vi "Persistent.vi"(8 "error in":T1, 10 "Persistent":bool, 11 "VISA Resource Name":refnum<visa-resource-name>="TCPIP0::10.0.0.1::7185::SOCKET") -> (0 "error out":T1, 3 "VISA Resource Name Out":refnum<visa-resource-name>)   [LabVIEW 2019]
uses:
  Persistent States.ctl
panel:
  out "Magnet Voltage retries":i16
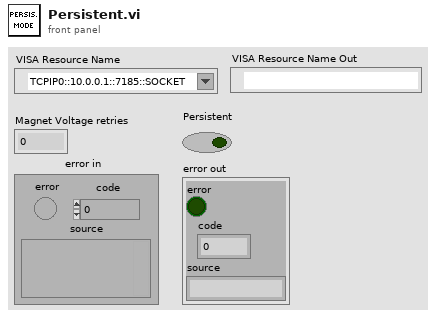
[diagram p1: front panel]
types:
  T1 = cluster{"error":bool, "code":i32, "source":string}
  T2 = typedef "Persistent States.ctl" = enum16{"Initialize", "Check Heater", "Check Mode Enter", "Check Magnet Voltage Enter", "Cool Switch", "Check Mode Exit", "Check Magnet Current Exit", "Heat Switch", "Stop"}
  T3 = enum16{"", "RAMPING", "HOLDING", "PAUSED", "MANUAL UP", "MANUAL DOWN", "ZEROING CURRENT", "QUENCH DETECTED", "AT ZERO", "HEATING SWITCH", "COOLING SWITCH", "EXTERNAL RAMPDOWN"}
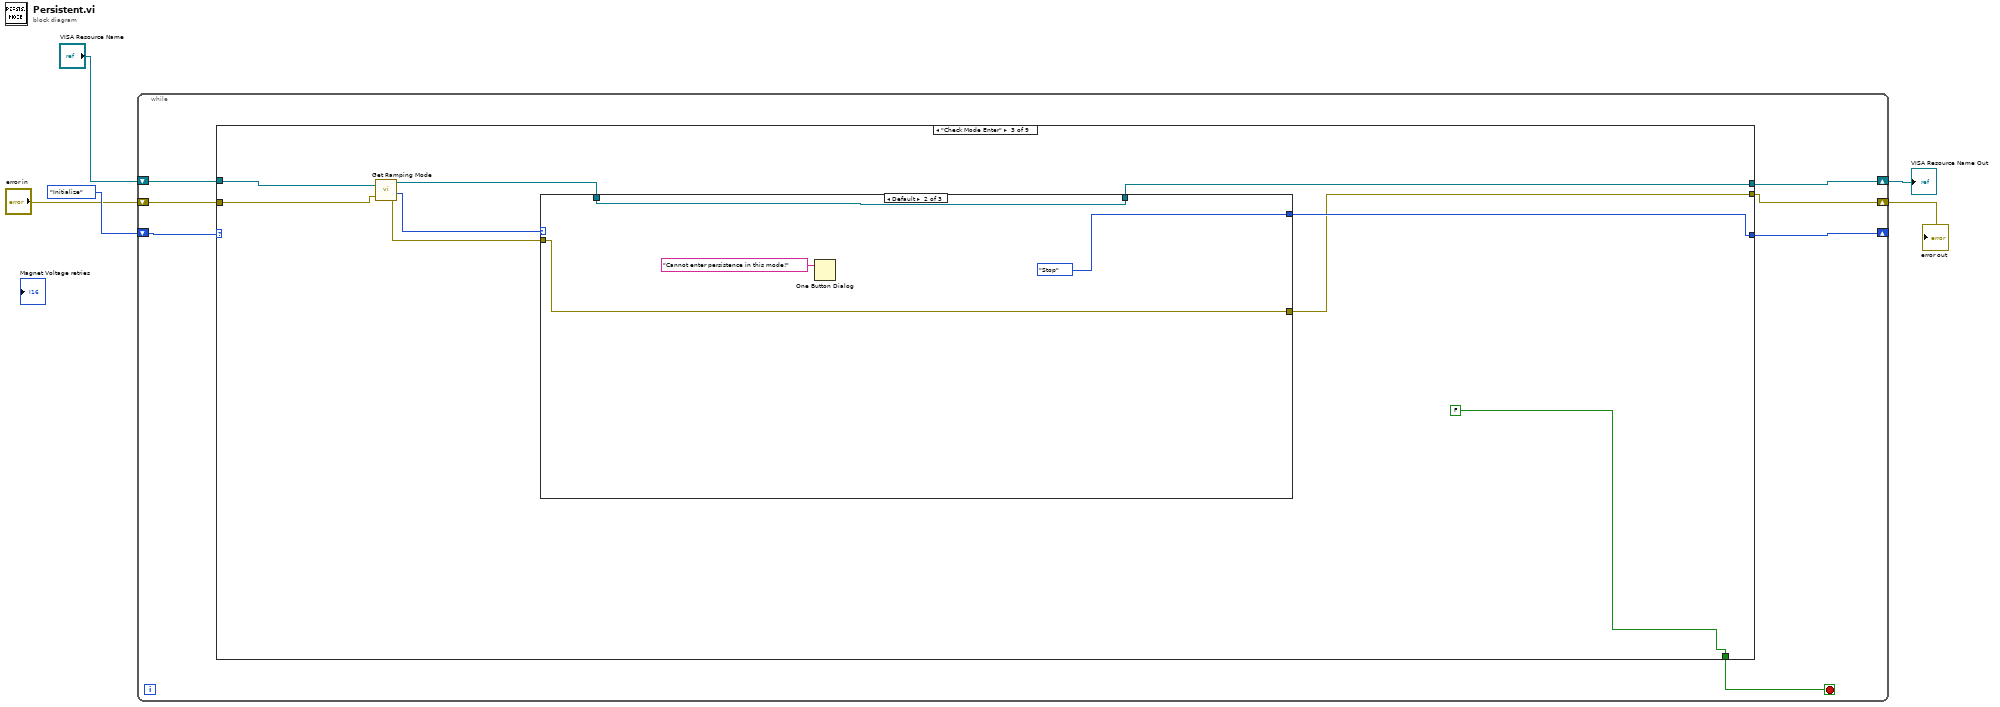
[diagram p0: block diagram]
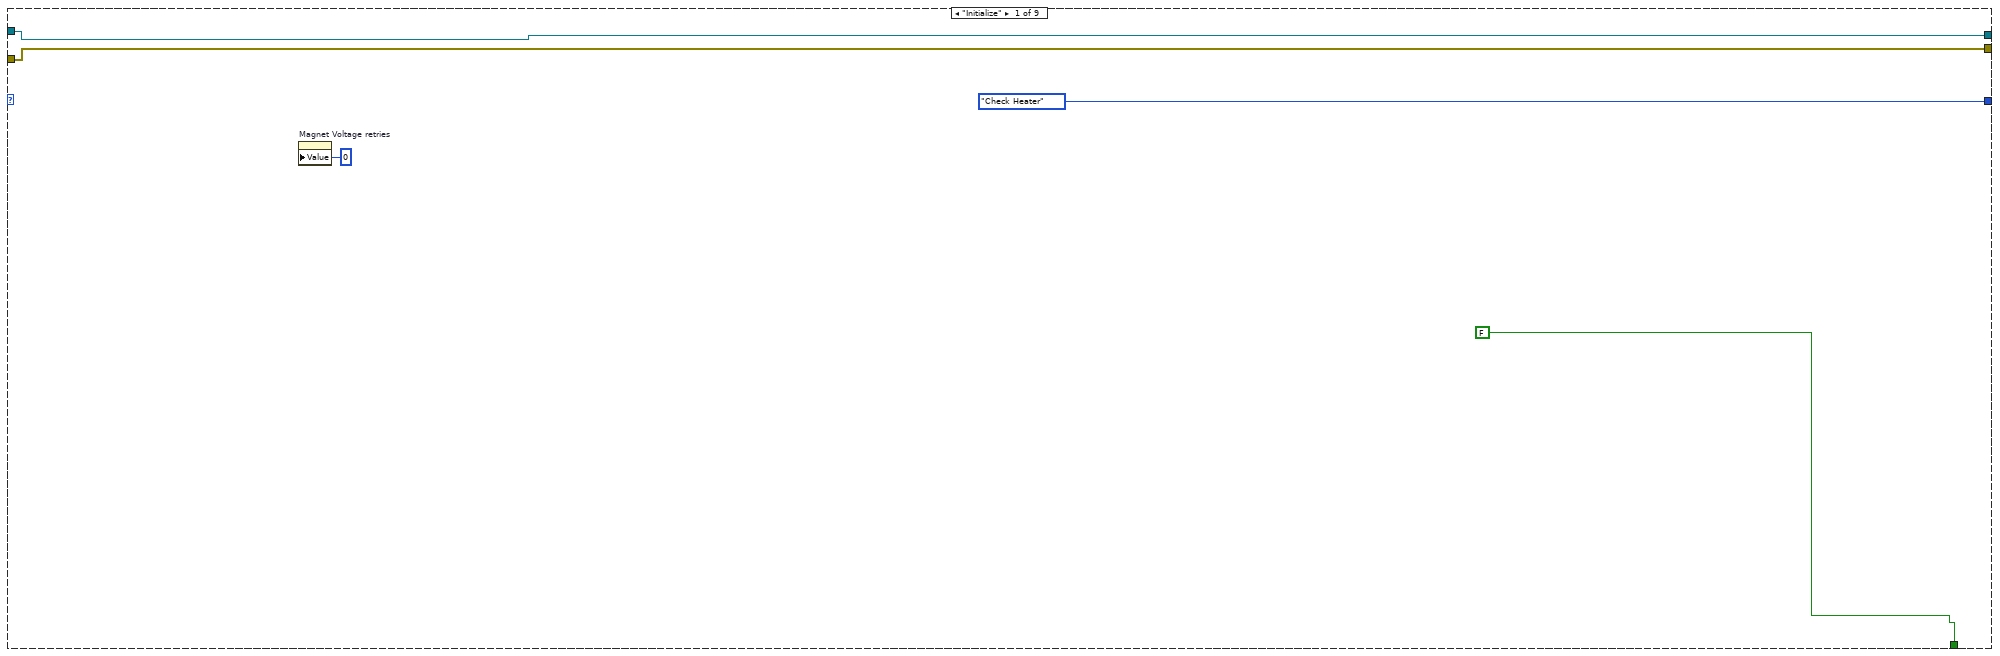
[diagram p2: hidden frame]
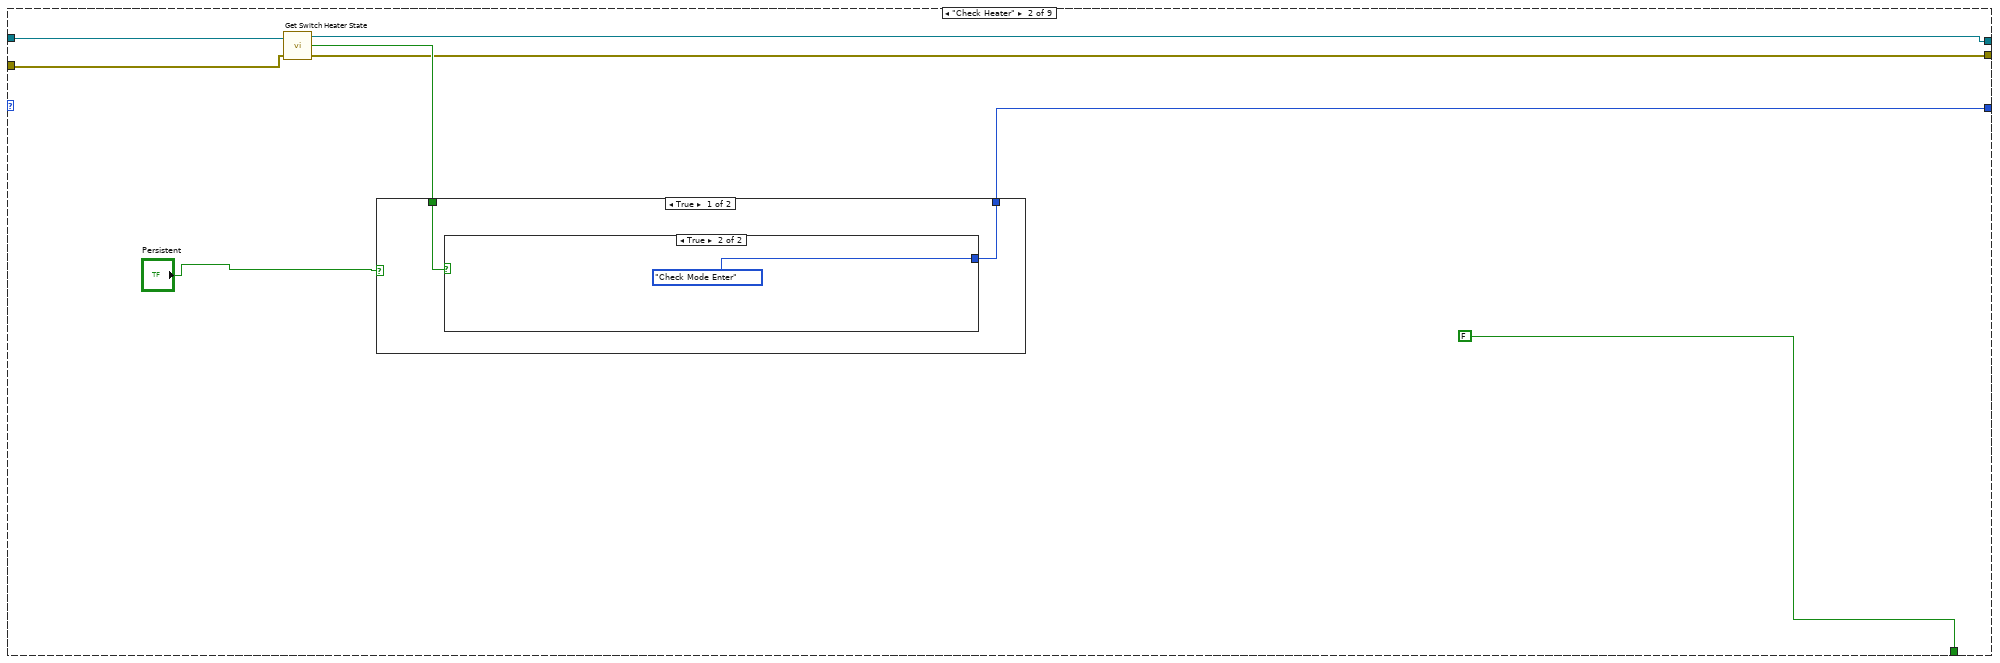
[diagram p3: hidden frame]
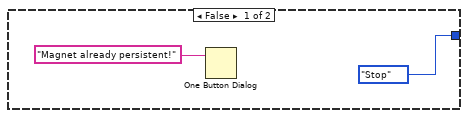
[diagram p4: hidden frame]
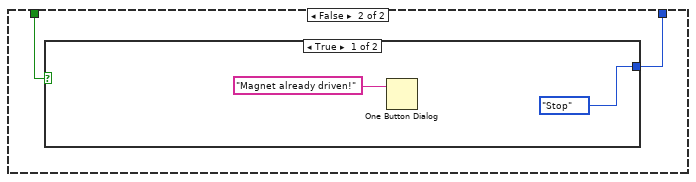
[diagram p5: hidden frame]
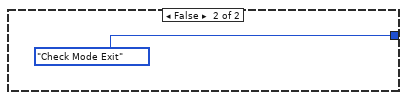
[diagram p6: hidden frame]
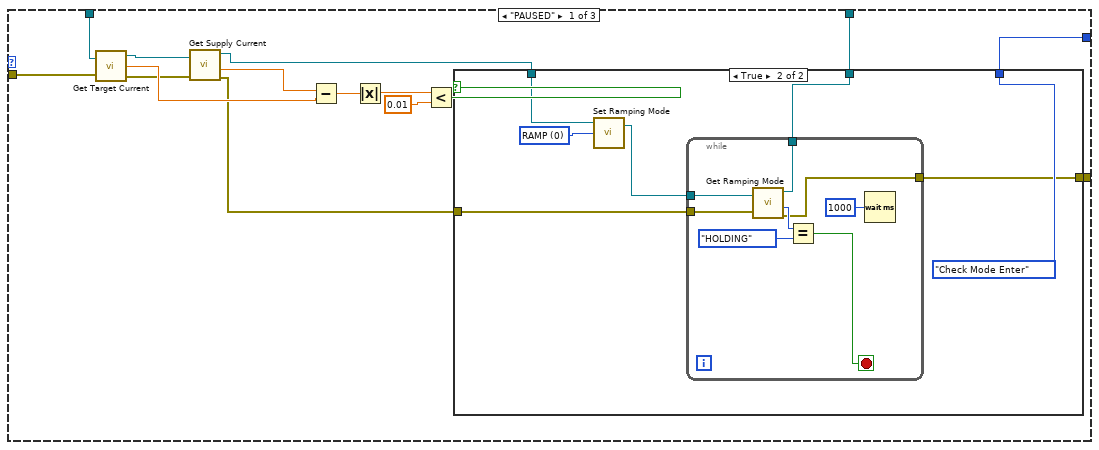
[diagram p7: hidden frame]
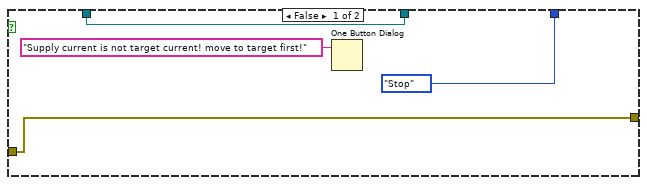
[diagram p8: hidden frame]
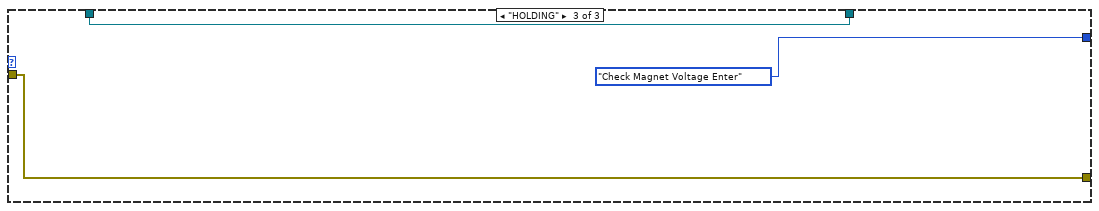
[diagram p9: hidden frame]
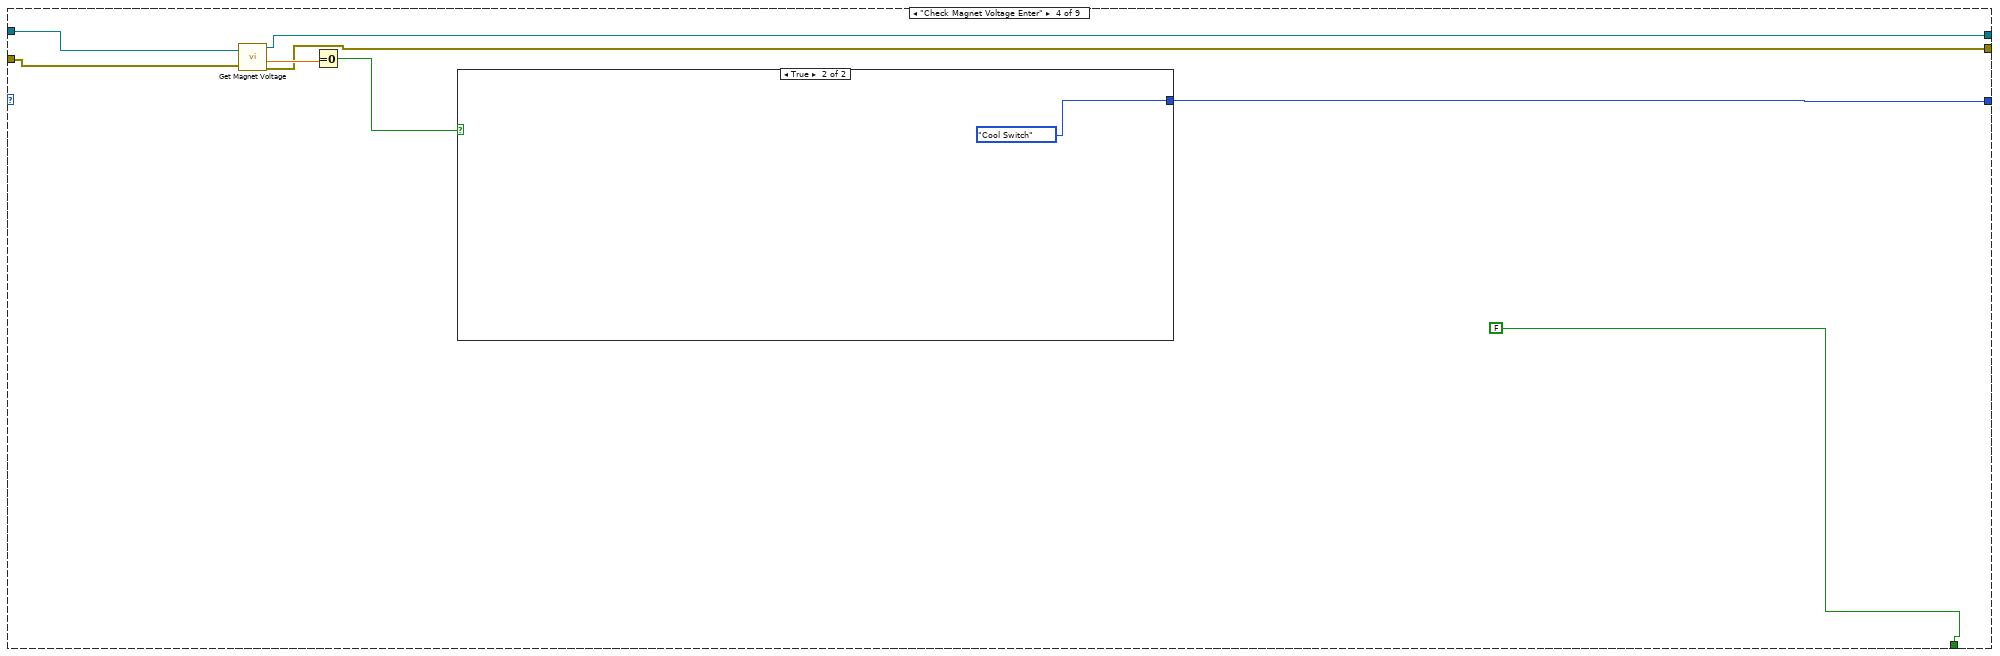
[diagram p10: hidden frame]
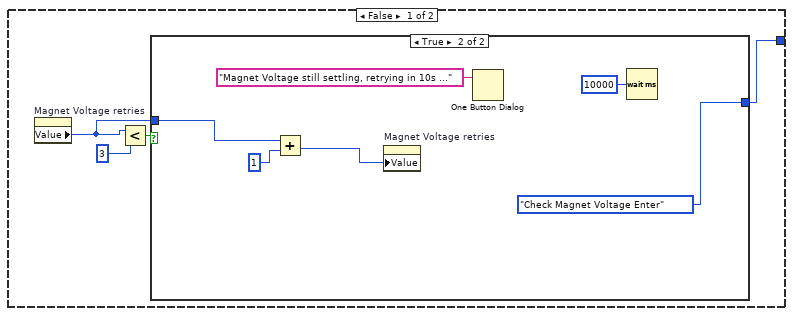
[diagram p11: hidden frame]
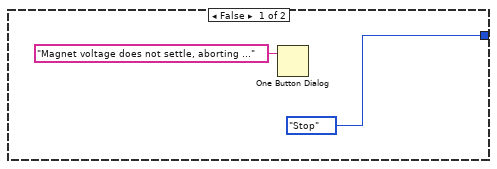
[diagram p12: hidden frame]
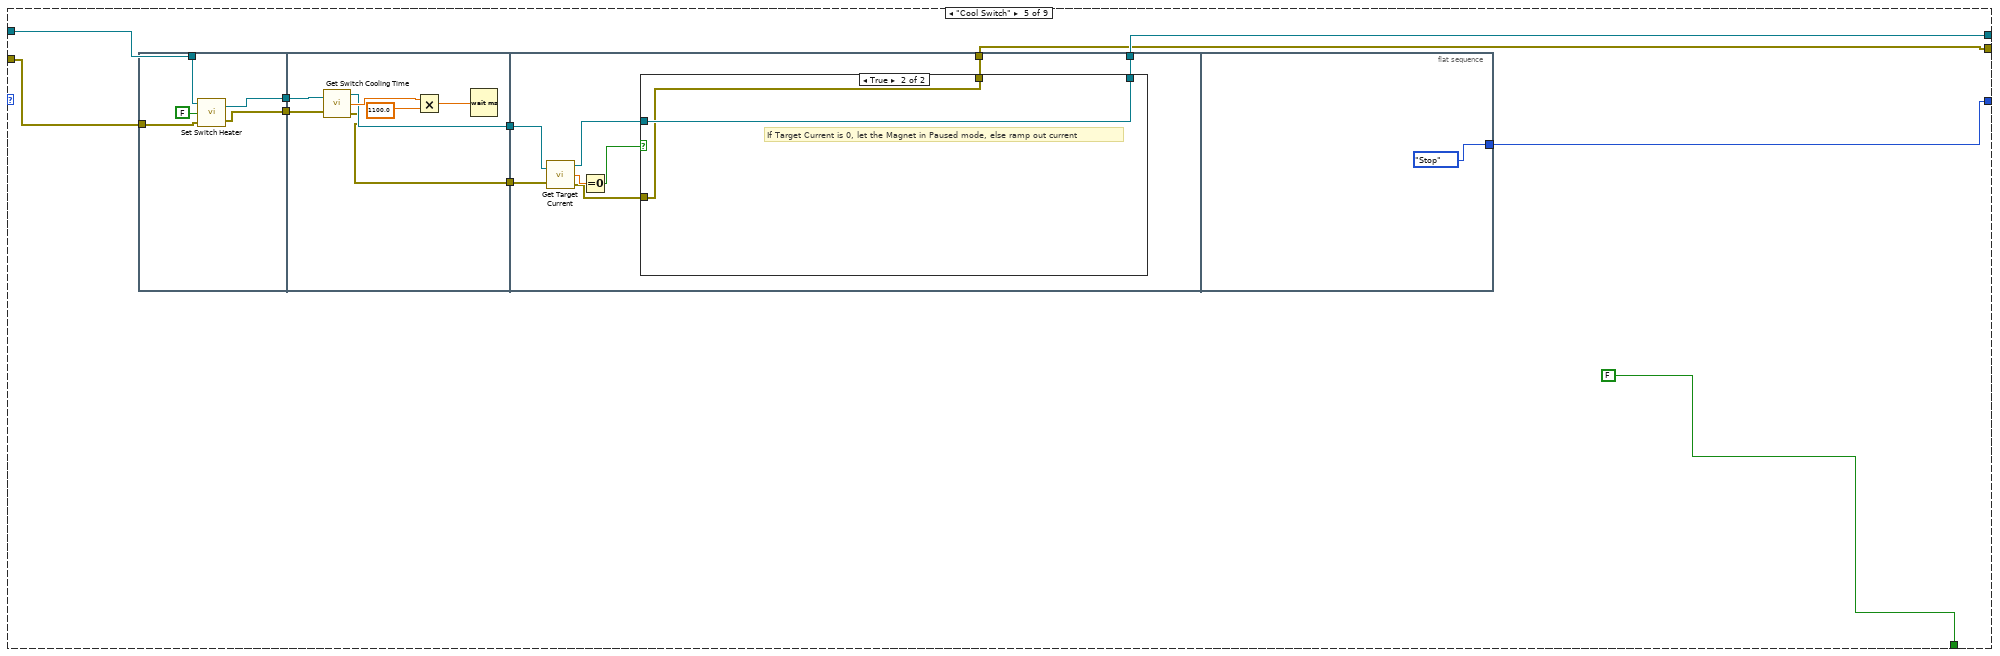
[diagram p13: hidden frame]
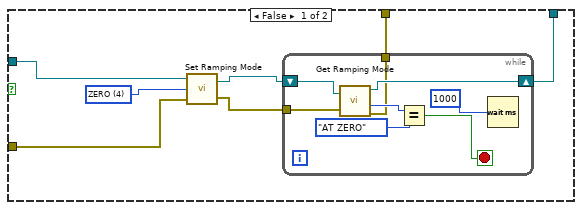
[diagram p14: hidden frame]
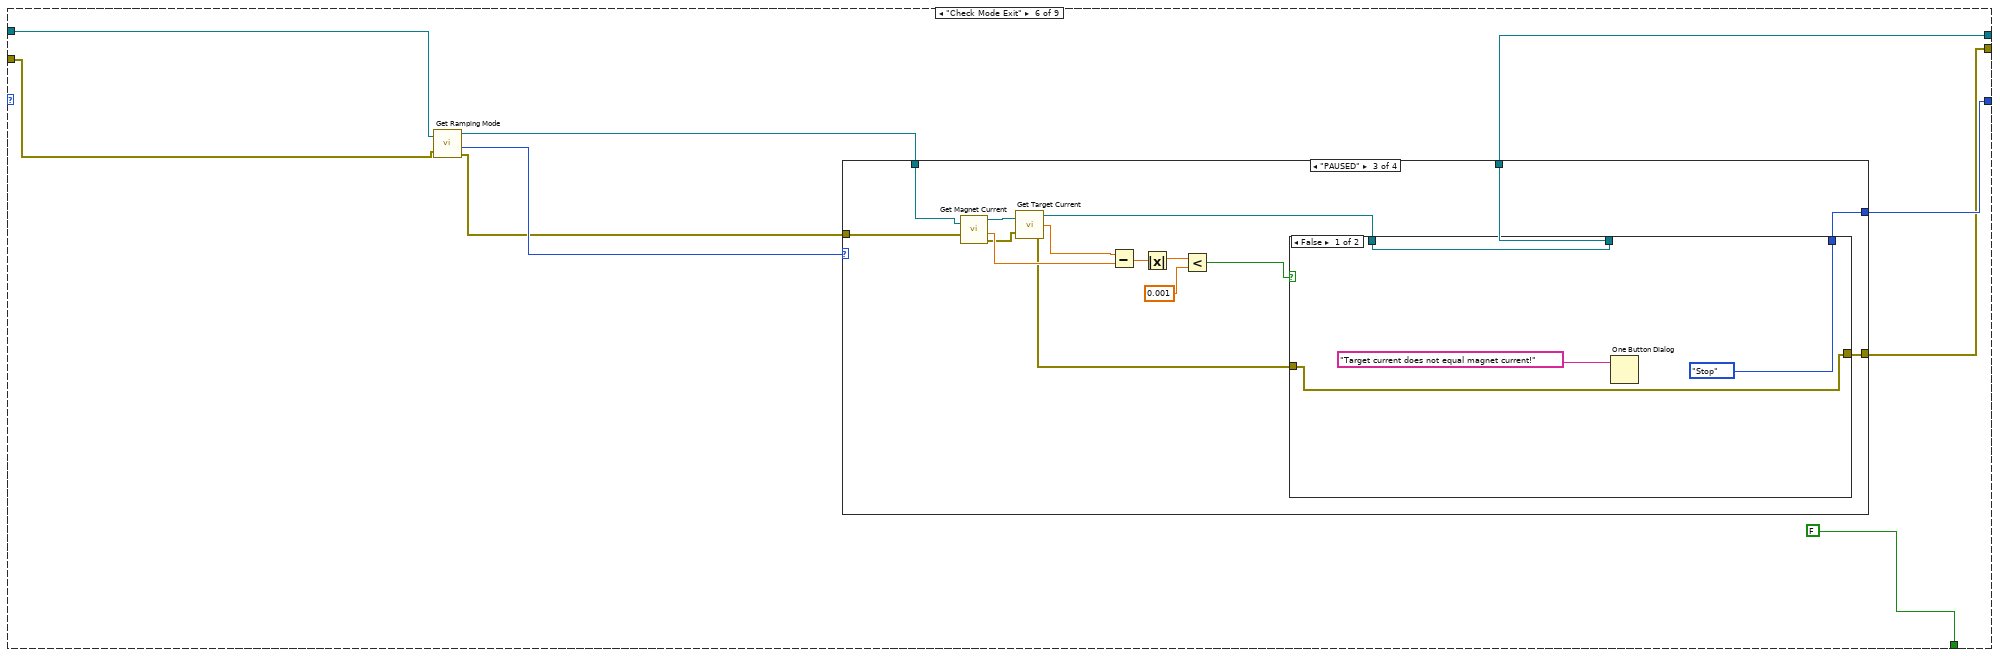
[diagram p15: hidden frame]
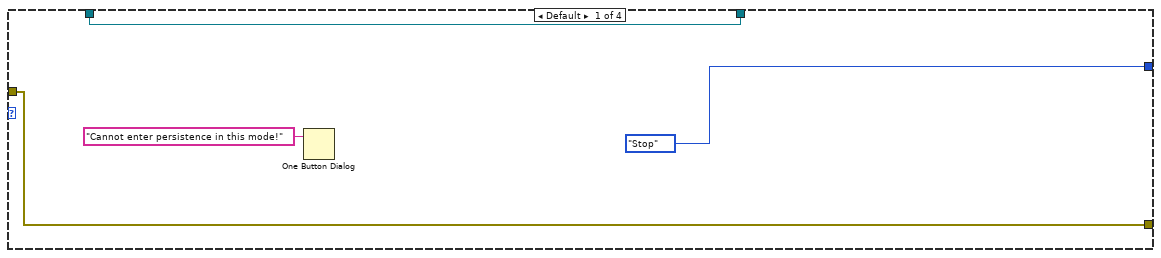
[diagram p16: hidden frame]
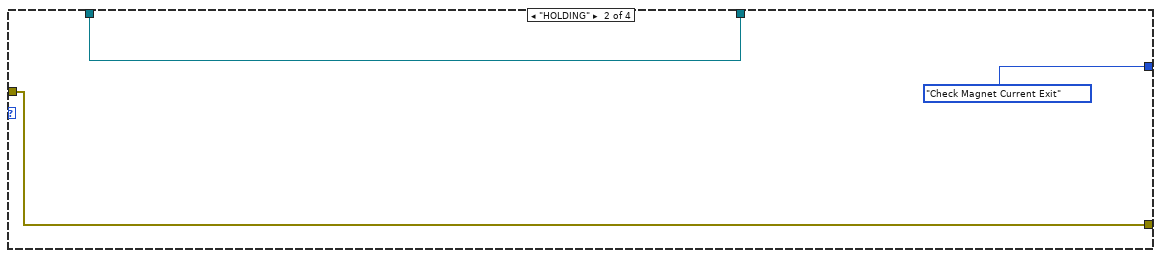
[diagram p17: hidden frame]
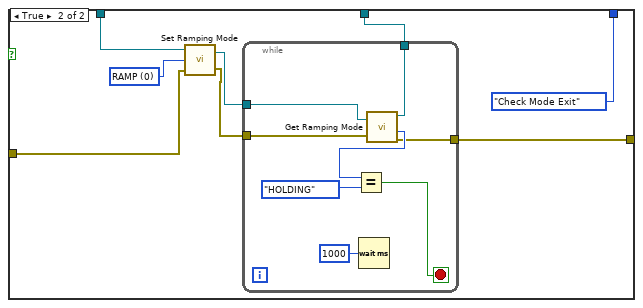
[diagram p18: hidden frame]
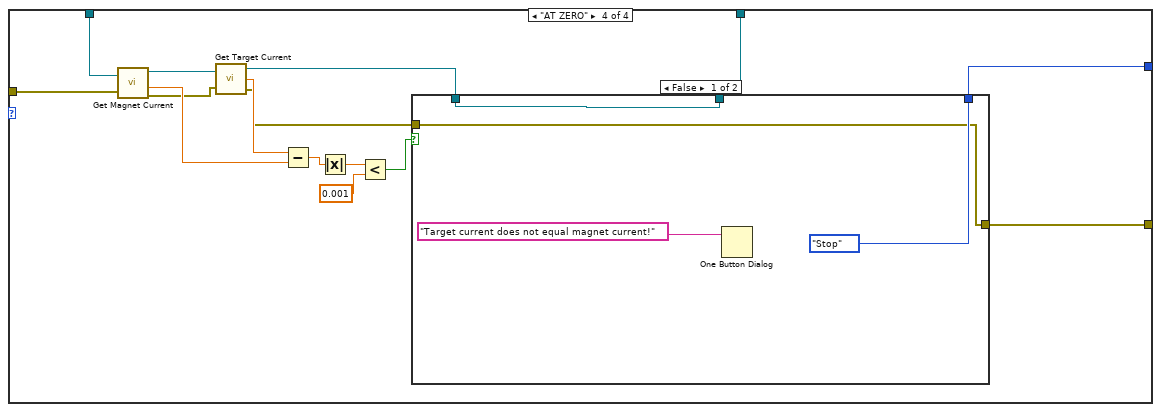
[diagram p19: hidden frame]
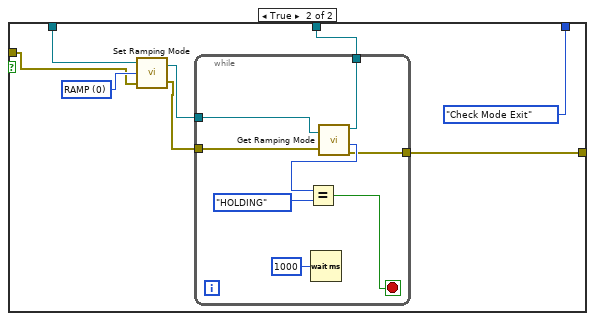
[diagram p20: hidden frame]
diagram:
  n1 = while {
    shift-right: [w10] -> _
    shift-left: Persistent_States."Initialize" -> [w12]
    shift-right: [w11] -> w3
    shift-left: "VISA Resource Name" -> [w9]
    shift-right: [w6] -> w1
    shift-left: "error in" -> [w7]
    stop <- w8 stop-if-true
    n2 = case shown="\"Check Mode Enter\"" w12 {
      tunnel: [w14 w24 w41 w92 w111 w159 w245 w262 w281] -> w11
      tunnel: [Persistent_States."Check Heater" w21 w40 w89 w113 w161 w246 w263 Persistent_States."Stop"] -> w10
      tunnel: w9 -> [w14 w25 w44 w93 w116 w163 w254 w265 w281]
      tunnel: [FALSE FALSE FALSE FALSE FALSE FALSE FALSE FALSE TRUE] -> w8
      tunnel: w7 -> [w13 w19 w38 w87 w110 w157 w243 w260 w279]
      tunnel: [w13 w18 w36 w86 w107 w155 w241 w258 w279] -> w6
      frame "Initialize" {
        n3 = property on="Magnet Voltage retries" class="DigNum (strict)"("Value"=i16 0 ("Magnet Voltage retries")) -> ()  [unwired: 2 in, 2 out]
      }
      frame "Check Heater" {
        n4 = call "Get Switch Heater State.vi"("error in"=w19, "VISA resource name"=w25) -> ("error out"=w18:T1, "Switch Heater state"=w22:bool, "VISA resource name out"=w24:refnum<visa-resource-name>)  [unwired: 1 in]
        n5 = case shown="True" "Persistent" {
          tunnel: w22 -> [w27 w32]
          tunnel: [w26 w31] -> w21
          frame True {
            n6 = case shown="True" w27 {
              tunnel: [Persistent_States."Stop" Persistent_States."Check Mode Enter"] -> w26
              frame False {
                n7 = One Button Dialog(message="Magnet already persistent!") -> ()  [unwired: 1 in, 1 out]
              }
              frame True {
              }
            }
          }
          frame False {
            n8 = case shown="True" w32 {
              tunnel: [Persistent_States."Stop" Persistent_States."Check Mode Exit"] -> w31
              frame True {
                n9 = One Button Dialog(message="Magnet already driven!") -> ()  [unwired: 1 in, 1 out]
              }
              frame False {
              }
            }
          }
        }
      }
      frame "Check Mode Enter" {
        n10 = call "Get Ramping Mode.vi"("VISA resource name"=w44, "error in"=w38) -> ("VISA resource name out"=w42:refnum<visa-resource-name>, "Ramping Mode"=w39:T3, "error out"=w37:T1)  [unwired: 1 out]
        n11 = case shown="Default" w39 {
          tunnel: [w51 Persistent_States."Stop" Persistent_States."Check Magnet Voltage Enter"] -> w40
          tunnel: w42 -> [w59 w80 w84]
          tunnel: [w49 w80 w84] -> w41
          tunnel: w37 -> [w48 w79 w83]
          tunnel: [w45 w79 w83] -> w36
          frame "PAUSED" {
            n12 = call "Get Target Current.vi"("VISA resource name"=w59, "error in"=w48) -> ("VISA resource name out"=w58:refnum<visa-resource-name>, "Target Current (A)"=w56:dbl, "error out"=w47:T1)
            n13 = call "Get Supply Current.vi"("VISA resource name"=w58, "error in"=w47) -> ("VISA resource name out"=w50:refnum<visa-resource-name>, "Supply Current (A)"=w57:dbl, "error out"=w46:T1)  [unwired: 1 out]
            n14 = Subtract(x=w57, y=w56) -> (x-y=w55:dbl)
            n15 = Absolute Value(x=w55) -> (abs(x)=w54:dbl)
            n16 = Less?(x=w54, y=0.01) -> (x < y?=w52:bool)
            n17 = case shown="True" w52 {
              tunnel: [Persistent_States."Stop" Persistent_States."Check Mode Enter"] -> w51
              tunnel: w50 -> [w61 w70]
              tunnel: [w61 w66] -> w49
              tunnel: w46 -> [w60 w65]
              tunnel: [w60 w64] -> w45
              frame False {
                n18 = One Button Dialog(message="Supply current is not target current! move to target first!") -> ()  [unwired: 1 in, 1 out]
              }
              frame True {
                w69 = u16 0 items=["RAMP", "PAUSE", "MANUAL UP", "MANUAL DOWN", "ZERO"] ("Ramping Mode")
                n19 = call "Set Ramping Mode.vi"("Ramping Mode"=w69, "VISA resource name"=w70) -> ("VISA resource name out"=w67:refnum<visa-resource-name>)  [unwired: 1 in, 1 out]
                n20 = while {
                  tunnel: w67 -> [w78]
                  tunnel: [w77] -> w66
                  tunnel: w65 -> [w72]
                  tunnel: [w71] -> w64
                  stop <- w74 stop-if-true
                  n21 = call "Get Ramping Mode.vi"("VISA resource name"=w78, "error in"=w72) -> ("VISA resource name out"=w77:refnum<visa-resource-name>, "Ramping Mode"=w76:T3, "error out"=w71:T1)  [unwired: 1 out]
                  n22 = Equal?(x=w76, y=T3."HOLDING") -> (x = y?=w74:bool)
                  n23 = Wait (ms)(milliseconds to wait=u32 1000) -> ()  [unwired: 1 out]
                }
              }
            }
          }
          frame Default {
            n24 = One Button Dialog(message="Cannot enter persistence in this mode!") -> ()  [unwired: 1 in, 1 out]
          }
          frame "HOLDING" {
          }
        }
      }
      frame "Check Magnet Voltage Enter" {
        n25 = call "Get Magnet Voltage.vi"("VISA resource name"=w93, "error in"=w87) -> ("VISA resource name out"=w92:refnum<visa-resource-name>, "Magnet Voltage (V)"=w91:dbl, "error out"=w86:T1)  [unwired: 1 out]
        n26 = Equal To 0?(x=w91) -> (x = 0?=w90:bool)
        n27 = case shown="True" w90 {
          tunnel: [w94 Persistent_States."Cool Switch"] -> w89
          frame False {
            n28 = property on="Magnet Voltage retries" class="DigNum (strict)"() -> ("Value"=w95:i16)  [unwired: 2 in, 2 out]
            n29 = Less?(x=w95, y=i16 3) -> (x < y?=w96:bool)
            n30 = case shown="True" w96 {
              tunnel: w95 -> [_ w105]
              tunnel: [Persistent_States."Stop" Persistent_States."Check Magnet Voltage Enter"] -> w94
              frame False {
                n31 = One Button Dialog(message="Magnet voltage does not settle, aborting ...") -> ()  [unwired: 1 in, 1 out]
              }
              frame True {
                n32 = Add(x=w105, y=i16 1) -> (x+y=w103:i16)
                n33 = property on="Magnet Voltage retries" class="DigNum (strict)"("Value"=w103) -> ()  [unwired: 2 in, 2 out]
                n34 = One Button Dialog(message="Magnet Voltage still settling, retrying in 10s ...") -> ()  [unwired: 1 in, 1 out]
                n35 = Wait (ms)(milliseconds to wait=u32 10000) -> ()  [unwired: 1 out]
              }
            }
          }
          frame True {
          }
        }
      }
      frame "Cool Switch" {
        n36 = flat-sequence {
          tunnel: w116 -> [w120]
          tunnel: [w119] -> w115
          tunnel: w110 -> [w118]
          tunnel: [w117] -> w109
          tunnel: w115 -> [w128]
          tunnel: [w124] -> w114
          tunnel: w109 -> [w123]
          tunnel: [w122] -> w108
          tunnel: w114 -> [w136]
          tunnel: [w132] -> w111
          tunnel: w108 -> [w131]
          tunnel: [w129] -> w107
          tunnel: [Persistent_States."Stop"] -> w113
          frame #0 {
            n37 = call "Set Switch Heater.vi"("error in"=w118, "Switch Heater Control"=FALSE, "VISA resource name"=w120) -> ("error out"=w117:T1, "VISA resource name out"=w119:refnum<visa-resource-name>)
          }
          frame #1 {
            n38 = call "Get Switch Cooling Time.vi"("VISA resource name"=w128, "error in"=w123) -> ("VISA resource name out"=w124:refnum<visa-resource-name>, "Switch Cooling Time (secs)"=w126:dbl, "error out"=w122:T1)
            n39 = Multiply(x=w126, y=1100.0) -> (x*y=w125:dbl)
            n40 = Wait (ms)(milliseconds to wait=w125) -> ()  [unwired: 1 out]
          }
          frame #2 {
            n41 = call "Get Target Current.vi"("VISA resource name"=w136, "error in"=w131) -> ("VISA resource name out"=w133:refnum<visa-resource-name>, "Target Current (A)"=w135:dbl, "error out"=w130:T1)
            n42 = Equal To 0?(x=w135) -> (x = 0?=w134:bool)
            n43 = case shown="True" w134 {
              tunnel: w133 -> [w142 w153]
              tunnel: [w140 w153] -> w132
              tunnel: w130 -> [w139 w152]
              tunnel: [w137 w152] -> w129
              frame False {
                w143 = u16 4 items=["RAMP", "PAUSE", "MANUAL UP", "MANUAL DOWN", "ZERO"] ("Ramping Mode")
                n44 = call "Set Ramping Mode.vi"("error in"=w139, "Ramping Mode"=w143, "VISA resource name"=w142) -> ("error out"=w138:T1, "VISA resource name out"=w141:refnum<visa-resource-name>)
                n45 = while {
                  shift-right: [w150] -> w140
                  shift-left: w141 -> [w151]
                  tunnel: w138 -> [w145]
                  tunnel: [w144] -> w137
                  stop <- w147 stop-if-true
                  n46 = call "Get Ramping Mode.vi"("VISA resource name"=w151, "error in"=w145) -> ("VISA resource name out"=w150:refnum<visa-resource-name>, "Ramping Mode"=w149:T3, "error out"=w144:T1)  [unwired: 1 out]
                  n47 = Equal?(x=w149, y=T3."AT ZERO") -> (x = y?=w147:bool)
                  n48 = Wait (ms)(milliseconds to wait=u32 1000) -> ()  [unwired: 1 out]
                }
              }
              frame True {
                # "If Target Current is 0, let the Magnet in Paused mode, else ramp out current"
              }
            }
          }
          frame #3 {
          }
        }
      }
      frame "Check Mode Exit" {
        n49 = call "Get Ramping Mode.vi"("VISA resource name"=w163, "error in"=w157) -> ("VISA resource name out"=w160:refnum<visa-resource-name>, "Ramping Mode"=w162:T3, "error out"=w156:T1)  [unwired: 1 out]
        n50 = case shown="\"PAUSED\"" w162 {
          tunnel: [Persistent_States."Stop" Persistent_States."Check Magnet Current Exit" w181 w217] -> w161
          tunnel: w160 -> [w165 w170 w185 w216]
          tunnel: [w165 w170 w182 w218] -> w159
          tunnel: w156 -> [w164 w168 w174 w209]
          tunnel: [w164 w168 w171 w206] -> w155
          frame Default {
            n51 = One Button Dialog(message="Cannot enter persistence in this mode!") -> ()  [unwired: 1 in, 1 out]
          }
          frame "HOLDING" {
          }
          frame "PAUSED" {
            n52 = call "Get Magnet Current.vi"("VISA resource name"=w185, "error in"=w174) -> ("VISA resource name out"=w184:refnum<visa-resource-name>, "Magnet Current (A)"=w179:dbl, "error out"=w173:T1)  [unwired: 1 out]
            n53 = call "Get Target Current.vi"("VISA resource name"=w184, "error in"=w173) -> ("VISA resource name out"=w183:refnum<visa-resource-name>, "Target Current (A)"=w180:dbl, "error out"=w172:T1)
            n54 = Subtract(x=w180, y=w179) -> (x-y=w178:dbl)
            n55 = Absolute Value(x=w178) -> (abs(x)=w177:dbl)
            n56 = Less?(x=w177, y=0.001) -> (x < y?=w175:bool)
            n57 = case shown="False" w175 {
              tunnel: w183 -> [w187 w197]
              tunnel: [w187 w194] -> w182
              tunnel: [Persistent_States."Stop" Persistent_States."Check Mode Exit"] -> w181
              tunnel: w172 -> [w186 w192]
              tunnel: [w186 w190] -> w171
              frame False {
                n58 = One Button Dialog(message="Target current does not equal magnet current!") -> ()  [unwired: 1 in, 1 out]
              }
              frame True {
                w196 = u16 0 items=["RAMP", "PAUSE", "MANUAL UP", "MANUAL DOWN", "ZERO"] ("Ramping Mode")
                n59 = call "Set Ramping Mode.vi"("error in"=w192, "Ramping Mode"=w196, "VISA resource name"=w197) -> ("error out"=w191:T1, "VISA resource name out"=w195:refnum<visa-resource-name>)
                n60 = while {
                  tunnel: w195 -> [w205]
                  tunnel: [w204] -> w194
                  tunnel: w191 -> [w199]
                  tunnel: [w198] -> w190
                  stop <- w201 stop-if-true
                  n61 = Wait (ms)(milliseconds to wait=u32 1000) -> ()  [unwired: 1 out]
                  n62 = call "Get Ramping Mode.vi"("VISA resource name"=w205, "error in"=w199) -> ("VISA resource name out"=w204:refnum<visa-resource-name>, "Ramping Mode"=w203:T3, "error out"=w198:T1)  [unwired: 1 out]
                  n63 = Equal?(x=w203, y=T3."HOLDING") -> (x = y?=w201:bool)
                }
              }
            }
          }
          frame "AT ZERO" {
            n64 = call "Get Magnet Current.vi"("VISA resource name"=w216, "error in"=w209) -> ("VISA resource name out"=w219:refnum<visa-resource-name>, "Magnet Current (A)"=w214:dbl, "error out"=w208:T1)  [unwired: 1 out]
            n65 = call "Get Target Current.vi"("VISA resource name"=w219, "error in"=w208) -> ("VISA resource name out"=w220:refnum<visa-resource-name>, "Target Current (A)"=w215:dbl, "error out"=w207:T1)
            n66 = Subtract(x=w215, y=w214) -> (x-y=w213:dbl)
            n67 = Absolute Value(x=w213) -> (abs(x)=w212:dbl)
            n68 = Less?(x=w212, y=0.001) -> (x < y?=w211:bool)
            n69 = case shown="False" w211 {
              tunnel: w220 -> [w222 w232]
              tunnel: [w222 w229] -> w218
              tunnel: [Persistent_States."Stop" Persistent_States."Check Mode Exit"] -> w217
              tunnel: w207 -> [w221 w227]
              tunnel: [w221 w225] -> w206
              frame False {
                n70 = One Button Dialog(message="Target current does not equal magnet current!") -> ()  [unwired: 1 in, 1 out]
              }
              frame True {
                w231 = u16 0 items=["RAMP", "PAUSE", "MANUAL UP", "MANUAL DOWN", "ZERO"] ("Ramping Mode")
                n71 = call "Set Ramping Mode.vi"("error in"=w227, "Ramping Mode"=w231, "VISA resource name"=w232) -> ("error out"=w226:T1, "VISA resource name out"=w230:refnum<visa-resource-name>)
                n72 = while {
                  tunnel: w230 -> [w240]
                  tunnel: [w239] -> w229
                  tunnel: w226 -> [w234]
                  tunnel: [w233] -> w225
                  stop <- w236 stop-if-true
                  n73 = Wait (ms)(milliseconds to wait=u32 1000) -> ()  [unwired: 1 out]
                  n74 = call "Get Ramping Mode.vi"("VISA resource name"=w240, "error in"=w234) -> ("VISA resource name out"=w239:refnum<visa-resource-name>, "Ramping Mode"=w238:T3, "error out"=w233:T1)  [unwired: 1 out]
                  n75 = Equal?(x=w238, y=T3."HOLDING") -> (x = y?=w236:bool)
                }
              }
            }
          }
        }
      }
      frame "Check Magnet Current Exit" {
        n76 = call "Get Magnet Current.vi"("VISA resource name"=w254, "error in"=w243) -> ("VISA resource name out"=w253:refnum<visa-resource-name>, "Magnet Current (A)"=w251:dbl, "error out"=w242:T1)  [unwired: 1 out]
        n77 = call "Get Supply Current.vi"("VISA resource name"=w253, "error in"=w242) -> ("VISA resource name out"=w245:refnum<visa-resource-name>, "Supply Current (A)"=w252:dbl, "error out"=w241:T1)  [unwired: 1 out]
        n78 = Subtract(x=w252, y=w251) -> (x-y=w250:dbl)
        n79 = Absolute Value(x=w250) -> (abs(x)=w249:dbl)
        n80 = Less?(x=w249, y=0.02) -> (x < y?=w247:bool)
        n81 = case shown="True" w247 {
          tunnel: [Persistent_States."Stop" Persistent_States."Heat Switch"] -> w246
          frame False {
            n82 = One Button Dialog(message="Supply current does not match magnet current!") -> ()  [unwired: 1 in, 1 out]
          }
          frame True {
          }
        }
      }
      frame "Heat Switch" {
        n83 = flat-sequence {
          tunnel: w265 -> [w270]
          tunnel: [w268] -> w264
          tunnel: w260 -> [w267]
          tunnel: [w266] -> w259
          tunnel: w264 -> [w277]
          tunnel: [w273] -> w262
          tunnel: w259 -> [w272]
          tunnel: [w271] -> w258
          tunnel: [Persistent_States."Stop"] -> w263
          frame #0 {
            n84 = call "Set Switch Heater.vi"("error in"=w267, "Switch Heater Control"=TRUE, "VISA resource name"=w270) -> ("error out"=w266:T1, "VISA resource name out"=w268:refnum<visa-resource-name>)
          }
          frame #1 {
            n85 = call "Get Switch Heating Time.vi"("VISA resource name"=w277, "error in"=w272) -> ("VISA resource name out"=w273:refnum<visa-resource-name>, "Switch Heating Time (secs)"=w276:dbl, "error out"=w271:T1)
            n86 = Multiply(x=w276, y=1100.0) -> (x*y=w274:dbl)
            n87 = Wait (ms)(milliseconds to wait=w274) -> ()  [unwired: 1 out]
          }
          frame #2 {
          }
        }
      }
      frame "Stop" {
      }
    }
  }
  "VISA Resource Name Out" <- w3
  "error out" <- w1
